vi "Adjust Mark10 Speed (1).vi"(8 "error in (no error)":errorcluster, 11 "Requested Speed":dbl) -> (0 "error out":errorcluster, 3 "Cmds":string[](array[string]))   [LabVIEW 2013]
uses:
  Controls/Mark10 Comm states.ctl
panel:
  in  "SpeedLimit":cluster{"Max":dbl, "Min":dbl}={"Max"=32.0, "Min"=0.0}
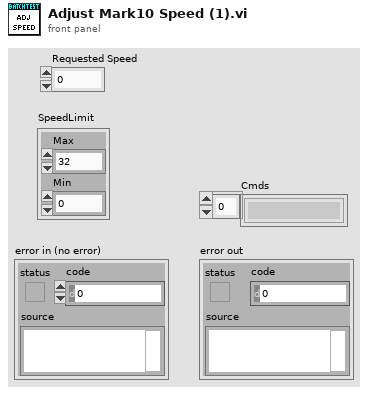
[diagram p1: front panel]
types:
  T1 = typedef "Mark10 Comm states.ctl" = enum16{"Open Session", "Get Reference", "Write Data", "Read Data", "Close Session"}
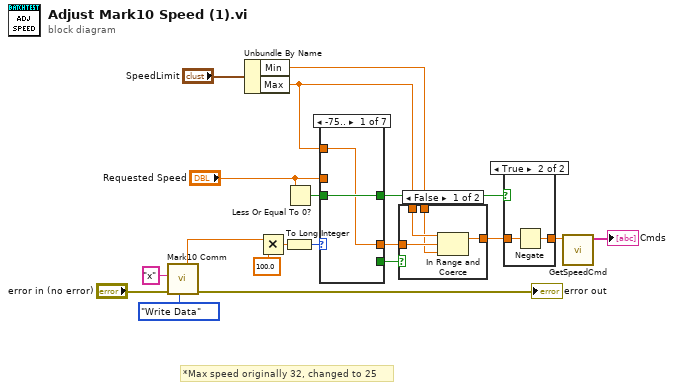
[diagram p0: block diagram]
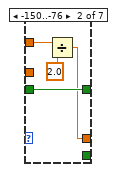
[diagram p4: hidden frame]
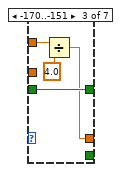
[diagram p5: hidden frame]
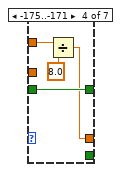
[diagram p6: hidden frame]
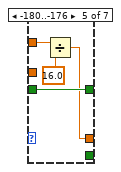
[diagram p7: hidden frame]
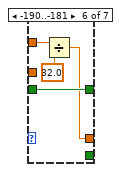
[diagram p8: hidden frame]
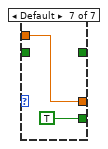
[diagram p9: hidden frame]
diagram:
  # "*Max speed originally 32, changed to 25"
  n1 = call "Mark10 Comm.vi"("Action"=Mark10_Comm_states."Write Data", "error in (no error)"="error in (no error)", "Write"="x") -> ("error out"=→"error out":errorcluster, "Position"=w15:dbl)  [unwired: 2 in, 5 out]
  n2 = Unbundle By Name("SpeedLimit") -> ("Min"=w1:dbl, "Max"=w2:dbl)
  n3 = Multiply(x=w15, y=100.0) -> (x*y=w12:dbl)
  n4 = To Long Integer(number=w12) -> (32bit integer=w14:i32)
  n5 = Less Or Equal To 0?(x="Requested Speed") -> (x <= 0?=w18:bool)
  n6 = case shown="-75.." w14 {
    tunnel: [w20 w22 w26 w30 w34 w38 w43] -> w6
    tunnel: "Requested Speed" -> [_ _ _ _ _ _ w43]
    tunnel: w18 -> [w21 w25 w29 w33 w37 w41 _]
    tunnel: [w21 w25 w29 w33 w37 w41 _] -> w19
    tunnel: [_ _ _ _ _ _ TRUE] -> w4
    tunnel: w2 -> [w20 w24 w27 w31 w35 w39 _]
    frame -75.. {
    }
    frame -150..-76 {
      n7 = Divide(x=w24, y=2.0) -> (x/y=w22:dbl)
    }
    frame -170..-151 {
      n8 = Divide(x=w27, y=4.0) -> (x/y=w26:dbl)
    }
    frame -175..-171 {
      n9 = Divide(x=w31, y=8.0) -> (x/y=w30:dbl)
    }
    frame -180..-176 {
      n10 = Divide(x=w35, y=16.0) -> (x/y=w34:dbl)
    }
    frame -190..-181 {
      n11 = Divide(x=w39, y=32.0) -> (x/y=w38:dbl)
    }
    frame Default {
    }
  }
  n12 = case shown="False" w4 {
    tunnel: w6 -> [w47 w48]
    tunnel: [w46 w48] -> w5
    tunnel: w2 -> [w45 _]
    tunnel: w1 -> [w44 _]
    frame False {
      n13 = In Range and Coerce(upper limit=w45, x=w47, lower limit=w44) -> (coerced(x)=w46:dbl)  [unwired: 1 out]
    }
    frame True {
    }
  }
  n14 = case shown="True" w19 {
    tunnel: w5 -> [w49 w51]
    tunnel: [w49 w50] -> w17
    frame False {
    }
    frame True {
      n15 = Negate(x=w51) -> (-x=w50:dbl)
    }
  }
  n16 = call "GetSpeedCmd.vi"("Speed"=w17) -> ("Cmds"=→"Cmds":string[])  [unwired: 10 in]
